vi "VMUI.vi"(10 "SubPanelRef":refnum<vi>, 11 "VariableManagerRef in":refnum<vi>) -> (3 "VariableManagerRef out":refnum<vi>)   [LabVIEW 2013]
doc: "The main user interface for VariableManager."
uses:
  VariableManager/VariableManager.lvclass
  VMUI.lvclass
  <vilib>/Utility/miscctls.llb/LVRowAndColumnUnsignedTypeDef.ctl
  SetListPrefs/SetListPrefs.lvclass/SetListPrefs.ctl
  <vilib>/Utility/miscctls.llb/LVRowAndColumnTypeDef.ctl
  Globals/PrefsGlobal.vi
  API/VariableManagerAPI.lvlib
  SetListPrefs/SetListPrefs.lvclass
panel:
  in  "VMUI":refnum<class "VMUI.lvclass">
  in  "Delete Variable":bool
  in  "Add Variable":bool
  in  "Edit Group":bool
  in  "Variable Group":u16(ring) items=["All"]
  in  "Detach":bool
  in  "Variables":string[][](table)
  in  "EvaluateSquenceValues":bool
  in  "Delete Sequence Index":bool
  in  "Add Sequence Index":bool
  in  "Sequence Indices":string[][](table)
  in  "Sequence Values":string[][](table) caption="Sequence Status"
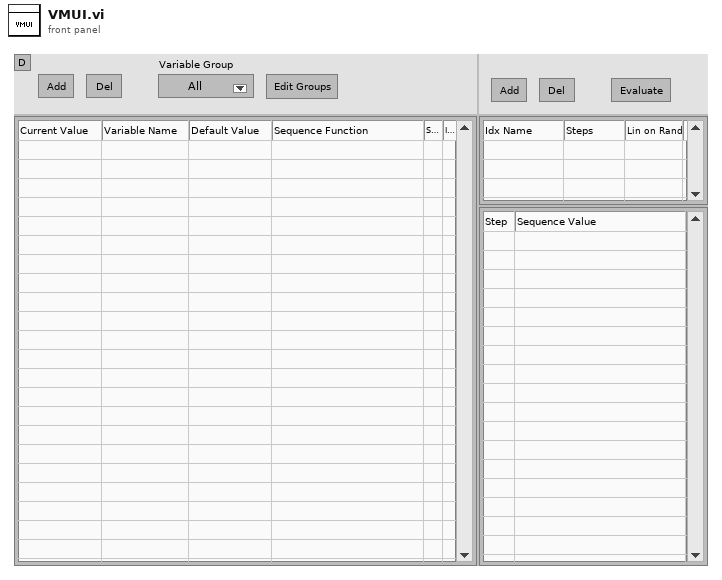
[diagram p1: front panel]
types:
  T1 = typedef "LVRowAndColumnUnsignedTypeDef.ctl" = cluster{"Row":u32, "Column":u32}
  T2 = typedef "LVRowAndColumnTypeDef.ctl" = cluster{"Row":i32, "Column":i32}
  T3 = cluster{"CtlRef":refnum<vi>, "OldVal":string[][], "NewVal":string[][]}
  T4 = typedef "LVPoint32TypeDef.ctl" = cluster{"Horizontal":i32, "Vertical":i32}
  T5 = cluster{"Shift":bool, "Ctrl":bool, "Alt":bool, "Cmd":bool, "Opt":bool}
  T6 = cluster{"CtlRef":refnum<vi>, "Coords":T4, "Button":u16, "Mods":cluster{"Double Click":bool, "Menu Key":bool}, "PlatMods":cluster{"Shift":bool, "Ctrl":bool, "Alt":bool, "Cmd":bool, "Opt":bool}}
  T7 = cluster{"Button":u16, "Mods":cluster{"Double Click":bool, "Menu Key":bool}, "PlatMods":cluster{"Shift":bool, "Ctrl":bool, "Alt":bool, "Cmd":bool, "Opt":bool}, "Discard?":bool}
  T8 = cluster{"CtlRef":refnum<vi>, "MenuRef":refnum<k9>, "Coords":T4, "SubObj":refnum<vi>}
  T9 = typedef "LVRectTypeDef.ctl" = cluster{"Left":i16, "Top":i16, "Right":i16, "Bottom":i16}
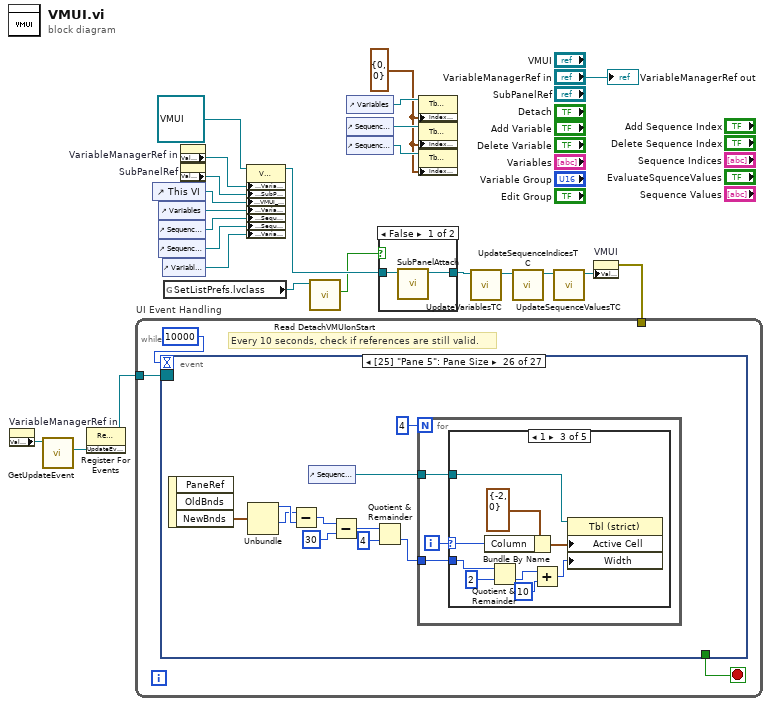
[diagram p0: block diagram]
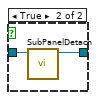
[diagram p2: hidden frame]
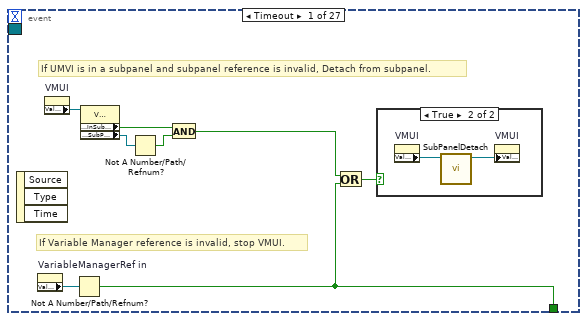
[diagram p3: hidden frame]
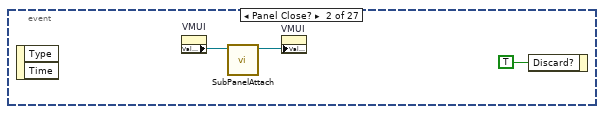
[diagram p5: hidden frame]
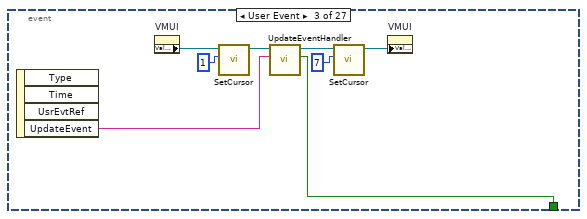
[diagram p6: hidden frame]
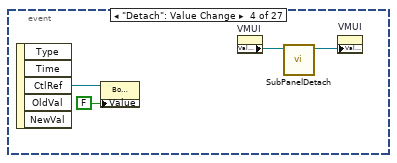
[diagram p7: hidden frame]
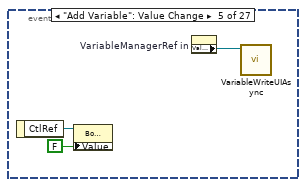
[diagram p8: hidden frame]
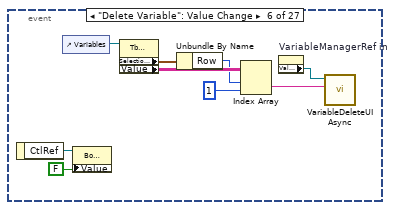
[diagram p9: hidden frame]
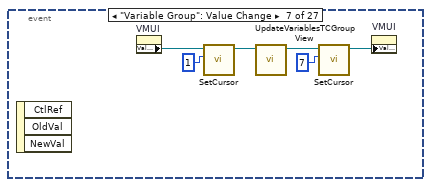
[diagram p10: hidden frame]
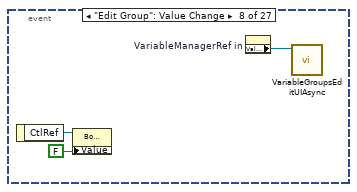
[diagram p11: hidden frame]
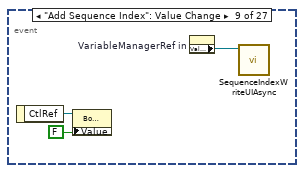
[diagram p12: hidden frame]
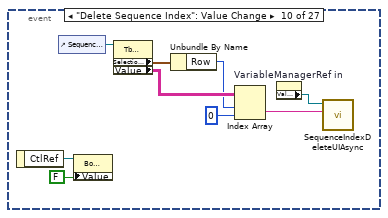
[diagram p13: hidden frame]
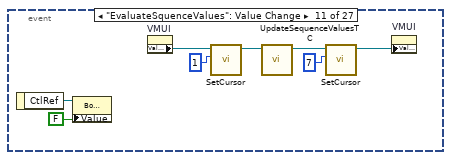
[diagram p14: hidden frame]
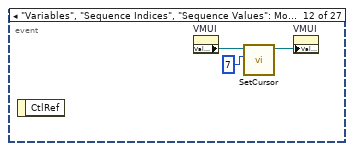
[diagram p15: hidden frame]
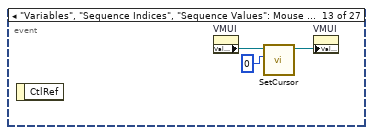
[diagram p16: hidden frame]
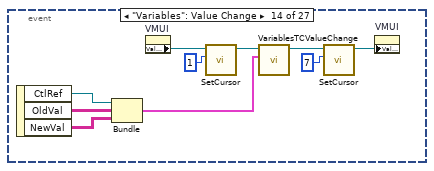
[diagram p17: hidden frame]
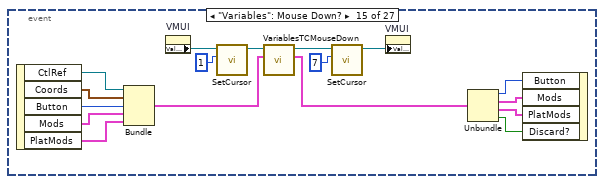
[diagram p18: hidden frame]
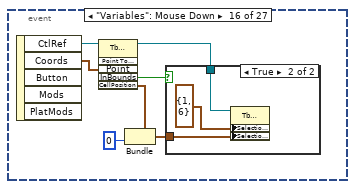
[diagram p19: hidden frame]
diagram:
  w4 = T1 {"Row"=0, "Column"=0} ("Index Values")
  n1 = property on="VariableManagerRef in" class="LVObjRef (strict)"() -> ("Value"=w15:refnum<vi>)  [unwired: 2 in, 2 out]
  n2 = call "GetUpdateEvent.vi"("VariableManagerRef in"=w15) -> ("UpdateEvent"=w14:refnum<user-event>)  [unwired: 8 in, 2 out]
  n3 = register-events(w14) -> (reference out=w13:refnum<event-registration>)  [unwired: 2 in, 1 out]
  n4 = control-ref of="This VI"() -> (w20:refnum<vi>)
  n5 = control-ref of="Variables"() -> (w19:refnum<vi>)
  n6 = control-ref of="Sequence Indices"() -> (w18:refnum<vi>)
  n7 = control-ref of="Sequence Values"() -> (w17:refnum<vi>)
  n8 = control-ref of="Variable Group"() -> (w16:refnum<vi>)
  n9 = global read "PrefsGlobal.vi" "SetListPrefs.lvclass"() -> (w2:refnum<class "SetListPrefs.lvclass">)
  n10 = property on="VariableManagerRef in" class="LVObjRef (strict)"() -> ("Value"=w22:refnum<vi>)  [unwired: 2 in, 2 out]
  n11 = property on="SubPanelRef" class="LVObjRef (strict)"() -> ("Value"=w21:refnum<vi>)  [unwired: 2 in, 2 out]
  n12 = property class="VMUI.lvclass"(reference=refnum<class "VMUI.lvclass"> refnum ("VMUI.lvclass"), "Accessors:VariableManagerRef"=w22, "Accessors:SubPanelRef"=w21, "Accessors:VMUI_VI_Ref"=w20, "Accessors:VariablesTCRef"=w19, "Accessors:SequenceIndicesTCRef"=w18, "Accessors:SequenceValuesTCRef"=w17, "Accessors:VariableGroupRingRef"=w16) -> (reference out=w12:refnum<class "VMUI.lvclass">)  [unwired: 1 in, 1 out]
  n13 = call "Read DetachVMUIonStart.vi"("SetListPrefs in"=w2) -> ("DetachVMUIonStart"=w1:bool)  [unwired: 8 in, 2 out]
  n14 = control-ref of="Variables"() -> (w7:refnum<vi>)
  n15 = control-ref of="Sequence Indices"() -> (w5:refnum<vi>)
  n16 = control-ref of="Sequence Values"() -> (w6:refnum<vi>)
  n17 = case shown="False" w1 {
    tunnel: w12 -> [w26 w27]
    tunnel: [w25 w28] -> w11
    frame False {
      n18 = call-dynamic "SubPanelAttach.vi"("VMUI in"=w26) -> ("VMUI out"=w25:refnum<class "VMUI.lvclass">)  [unwired: 9 in, 1 out]
    }
    frame True {
      n19 = call-dynamic "SubPanelDetach.vi"("VMUI in"=w27) -> ("VMUI out"=w28:refnum<class "VMUI.lvclass">)  [unwired: 9 in, 1 out]
    }
  }
  n20 = property class="Tbl (strict)"(reference=w7, "Index Values"=w4) -> ()  [unwired: 1 in, 2 out]
  n21 = property class="Tbl (strict)"(reference=w5, "Index Values"=w4) -> ()  [unwired: 1 in, 2 out]
  n22 = property class="Tbl (strict)"(reference=w6, "Index Values"=w4) -> ()  [unwired: 1 in, 2 out]
  n23 = call-dynamic "UpdateVariablesTC.vi"("VMUI in"=w11) -> ("VMUI out"=w10:refnum<class "VMUI.lvclass">)  [unwired: 9 in, 1 out]
  n24 = call-dynamic "UpdateSequenceIndicesTC.vi"("VMUI in"=w10) -> ("VMUI out"=w9:refnum<class "VMUI.lvclass">)  [unwired: 9 in, 1 out]
  n25 = call-dynamic "UpdateSequenceValuesTC.vi"("VMUI in"=w9) -> ("VMUI out"=w8:refnum<class "VMUI.lvclass">)  [unwired: 9 in, 1 out]
  n26 = property on="VMUI" class="LVClassControl (strict)"("Value"=w8) -> (error out=w3:errorcluster)  [unwired: 2 in, 1 out]
  n27 = while "UI Event Handling" {
    tunnel: w13 -> [w31]
    tunnel: w3 -> [_]
    stop <- w30 stop-if-true
    # "Every 10 seconds, check if references are still valid."
    n28 = event shown="[25] \"Pane 5\": Pane Size" {
      selector: w31 -> [_ _ _ _ _ _ _ _ _ _ _ _ _ _ _ _ _ _ _ _ _ _ _ _ _ _ _]
      dyn-events: _ -> [_ _ _ _ _ _ _ _ _ _ _ _ _ _ _ _ _ _ _ _ _ _ _ _ _ _ _]
      timeout: 10000 -> [_ _ _ _ _ _ _ _ _ _ _ _ _ _ _ _ _ _ _ _ _ _ _ _ _ _ _]
      tunnel: [w32 _ w51 _ _ _ _ _ _ _ _ _ _ _ _ _ _ _ _ _ _ _ _ _ _ _ _] -> w30
      event Timeout {
        # "If UMVI is in a subpanel and subpanel reference is invalid, Detach from subpanel."
        # "If Variable Manager reference is invalid, stop VMUI."
        n29 = event-data() -> ()  [unwired: 1 in, 3 out]
        n30 = property on="VariableManagerRef in" class="LVObjRef (strict)"() -> ("Value"=w39:refnum<vi>)  [unwired: 2 in, 2 out]
        n31 = property on="VMUI" class="LVClassControl (strict)"() -> ("Value"=w38:refnum<class "VMUI.lvclass">)  [unwired: 2 in, 2 out]
        n32 = Not A Number/Path/Refnum?(number/path/refnum=w39) -> (NaN/Path/Refnum?=w32:bool)
        n33 = property class="VMUI.lvclass"(reference=w38) -> ("Accessors:InSubPanel"=w36:bool, "Accessors:SubPanelRef"=w37:refnum<vi>)  [unwired: 1 in, 2 out]
        n34 = Not A Number/Path/Refnum?(number/path/refnum=w37) -> (NaN/Path/Refnum?=w35:bool)
        n35 = And(x=w36, y=w35) -> (x .and. y?=w33:bool)
        n36 = Or(x=w33, y=w32) -> (x .or. y?=w34:bool)
        n37 = case shown="True" w34 {
          frame False {
          }
          frame True {
            n38 = property on="VMUI" class="LVClassControl (strict)"() -> ("Value"=w41:refnum<class "VMUI.lvclass">)  [unwired: 2 in, 2 out]
            n39 = call-dynamic "SubPanelDetach.vi"("VMUI in"=w41) -> ("VMUI out"=w40:refnum<class "VMUI.lvclass">)  [unwired: 9 in, 1 out]
            n40 = property on="VMUI" class="LVClassControl (strict)"("Value"=w40) -> ()  [unwired: 2 in, 2 out]
          }
        }
      }
      event Panel Close? {
        n41 = event-data() -> ()  [unwired: 1 in, 2 out]
        n42 = property on="VMUI" class="LVClassControl (strict)"() -> ("Value"=w43:refnum<class "VMUI.lvclass">)  [unwired: 2 in, 2 out]
        n43 = call-dynamic "SubPanelAttach.vi"("VMUI in"=w43) -> ("VMUI out"=w42:refnum<class "VMUI.lvclass">)  [unwired: 9 in, 1 out]
        n44 = property on="VMUI" class="LVClassControl (strict)"("Value"=w42) -> ()  [unwired: 2 in, 2 out]
        n45 = event-data("Discard?"=TRUE) -> ()  [unwired: 1 in, 1 out]
      }
      event User Event {
        n46 = event-data() -> ("UpdateEvent"=w52:string)  [unwired: 1 in, 3 out]
        n47 = property on="VMUI" class="LVClassControl (strict)"() -> ("Value"=w48:refnum<class "VMUI.lvclass">)  [unwired: 2 in, 2 out]
        n48 = call-dynamic "SetCursor.vi"("icon"=u16 1, "VMUI in"=w48) -> ("VMUI out"=w47:refnum<class "VMUI.lvclass">)  [unwired: 8 in, 1 out]
        n49 = call-dynamic "UpdateEventHandler.vi"("UpdateEvent"=w52, "VMUI in"=w47) -> ("Stop"=w51:bool, "VMUI out"=w46:refnum<class "VMUI.lvclass">)  [unwired: 7 in, 1 out]
        n50 = call-dynamic "SetCursor.vi"("icon"=u16 7, "VMUI in"=w46) -> ("VMUI out"=w45:refnum<class "VMUI.lvclass">)  [unwired: 8 in, 1 out]
        n51 = property on="VMUI" class="LVClassControl (strict)"("Value"=w45) -> ()  [unwired: 2 in, 2 out]
      }
      event "Detach": Value Change {
        n52 = event-data() -> ("CtlRef"=w55:refnum<vi>)  [unwired: 1 in, 4 out]
        n53 = property class="Bool (strict)"(reference=w55, "Value"=FALSE) -> ()  [unwired: 1 in, 2 out]
        n54 = property on="VMUI" class="LVClassControl (strict)"() -> ("Value"=w54:refnum<class "VMUI.lvclass">)  [unwired: 2 in, 2 out]
        n55 = call-dynamic "SubPanelDetach.vi"("VMUI in"=w54) -> ("VMUI out"=w53:refnum<class "VMUI.lvclass">)  [unwired: 9 in, 1 out]
        n56 = property on="VMUI" class="LVClassControl (strict)"("Value"=w53) -> ()  [unwired: 2 in, 2 out]
      }
      event "Add Variable": Value Change {
        n57 = event-data() -> ("CtlRef"=w59:refnum<vi>)  [unwired: 1 in]
        n58 = property class="Bool (strict)"(reference=w59, "Value"=FALSE) -> ()  [unwired: 1 in, 2 out]
        n59 = property on="VariableManagerRef in" class="LVObjRef (strict)"() -> ("Value"=w57:refnum<vi>)  [unwired: 2 in, 2 out]
        n60 = call "VariableWriteUIAsync.vi"("VariableManagerRef in"=w57) -> ()  [unwired: 11 in]
      }
      event "Delete Variable": Value Change {
        n61 = event-data() -> ("CtlRef"=w68:refnum<vi>)  [unwired: 1 in]
        n62 = control-ref of="Variables"() -> (w62:refnum<vi>)
        n63 = property class="Bool (strict)"(reference=w68, "Value"=FALSE) -> ()  [unwired: 1 in, 2 out]
        n64 = property class="Tbl (strict)"(reference=w62) -> ("Selection Start"=w66:T2, "Value"=w65:string[][])  [unwired: 1 in, 2 out]
        n65 = Unbundle By Name(w66) -> ("Row"=w64:i32)
        n66 = Index Array(array=w65, index (row)=w64, index (col)=1 ("disabled index (col)")) -> (element=w60:string)
        n67 = property on="VariableManagerRef in" class="LVObjRef (strict)"() -> ("Value"=w61:refnum<vi>)  [unwired: 2 in, 2 out]
        n68 = call "VariableDeleteUIAsync.vi"("VariableName"=w60, "VariableManagerRef in"=w61) -> ()  [unwired: 10 in]
      }
      event "Variable Group": Value Change {
        n69 = event-data() -> ()  [unwired: 1 in, 3 out]
        n70 = property on="VMUI" class="LVClassControl (strict)"() -> ("Value"=w72:refnum<class "VMUI.lvclass">)  [unwired: 2 in, 2 out]
        n71 = call-dynamic "SetCursor.vi"("icon"=u16 1, "VMUI in"=w72) -> ("VMUI out"=w71:refnum<class "VMUI.lvclass">)  [unwired: 8 in, 1 out]
        n72 = call-dynamic "UpdateVariablesTCGroupView.vi"("VMUI in"=w71) -> ("VMUI out"=w70:refnum<class "VMUI.lvclass">)  [unwired: 9 in, 1 out]
        n73 = call-dynamic "SetCursor.vi"("icon"=u16 7, "VMUI in"=w70) -> ("VMUI out"=w69:refnum<class "VMUI.lvclass">)  [unwired: 8 in, 1 out]
        n74 = property on="VMUI" class="LVClassControl (strict)"("Value"=w69) -> ()  [unwired: 2 in, 2 out]
      }
      event "Edit Group": Value Change {
        n75 = event-data() -> ("CtlRef"=w77:refnum<vi>)  [unwired: 1 in]
        n76 = property class="Bool (strict)"(reference=w77, "Value"=FALSE) -> ()  [unwired: 1 in, 2 out]
        n77 = property on="VariableManagerRef in" class="LVObjRef (strict)"() -> ("Value"=w75:refnum<vi>)  [unwired: 2 in, 2 out]
        n78 = call "VariableGroupsEditUIAsync.vi"("VariableManagerRef in"=w75) -> ()  [unwired: 11 in]
      }
      event "Add Sequence Index": Value Change {
        n79 = event-data() -> ("CtlRef"=w80:refnum<vi>)  [unwired: 1 in]
        n80 = property class="Bool (strict)"(reference=w80, "Value"=FALSE) -> ()  [unwired: 1 in, 2 out]
        n81 = property on="VariableManagerRef in" class="LVObjRef (strict)"() -> ("Value"=w78:refnum<vi>)  [unwired: 2 in, 2 out]
        n82 = call "SequenceIndexWriteUIAsync.vi"("VariableManagerRef in"=w78) -> ()  [unwired: 11 in]
      }
      event "Delete Sequence Index": Value Change {
        n83 = event-data() -> ("CtlRef"=w89:refnum<vi>)  [unwired: 1 in]
        n84 = control-ref of="Sequence Indices"() -> (w83:refnum<vi>)
        n85 = property class="Bool (strict)"(reference=w89, "Value"=FALSE) -> ()  [unwired: 1 in, 2 out]
        n86 = property class="Tbl (strict)"(reference=w83) -> ("Selection Start"=w87:T2, "Value"=w86:string[][])  [unwired: 1 in, 2 out]
        n87 = Unbundle By Name(w87) -> ("Row"=w85:i32)
        n88 = Index Array(array=w86, index (row)=w85, index (col)=0 ("disabled index (col)")) -> (element=w81:string)
        n89 = property on="VariableManagerRef in" class="LVObjRef (strict)"() -> ("Value"=w82:refnum<vi>)  [unwired: 2 in, 2 out]
        n90 = call "SequenceIndexDeleteUIAsync.vi"("SequenceIndexName"=w81, "VariableManagerRef in"=w82) -> ()  [unwired: 10 in]
      }
      event "EvaluateSquenceValues": Value Change {
        n91 = event-data() -> ("CtlRef"=w97:refnum<vi>)  [unwired: 1 in]
        n92 = property class="Bool (strict)"(reference=w97, "Value"=FALSE) -> ()  [unwired: 1 in, 2 out]
        n93 = property on="VMUI" class="LVClassControl (strict)"() -> ("Value"=w93:refnum<class "VMUI.lvclass">)  [unwired: 2 in, 2 out]
        n94 = call-dynamic "SetCursor.vi"("icon"=u16 1, "VMUI in"=w93) -> ("VMUI out"=w92:refnum<class "VMUI.lvclass">)  [unwired: 8 in, 1 out]
        n95 = call-dynamic "UpdateSequenceValuesTC.vi"("VMUI in"=w92) -> ("VMUI out"=w91:refnum<class "VMUI.lvclass">)  [unwired: 9 in, 1 out]
        n96 = call-dynamic "SetCursor.vi"("icon"=u16 7, "VMUI in"=w91) -> ("VMUI out"=w90:refnum<class "VMUI.lvclass">)  [unwired: 8 in, 1 out]
        n97 = property on="VMUI" class="LVClassControl (strict)"("Value"=w90) -> ()  [unwired: 2 in, 2 out]
      }
      event "Variables", "Sequence Indices", "Sequence Values": Mouse Enter {
        n98 = event-data() -> ()  [unwired: 1 in, 1 out]
        n99 = property on="VMUI" class="LVClassControl (strict)"() -> ("Value"=w100:refnum<class "VMUI.lvclass">)  [unwired: 2 in, 2 out]
        n100 = call-dynamic "SetCursor.vi"("icon"=u16 7, "VMUI in"=w100) -> ("VMUI out"=w99:refnum<class "VMUI.lvclass">)  [unwired: 8 in, 1 out]
        n101 = property on="VMUI" class="LVClassControl (strict)"("Value"=w99) -> ()  [unwired: 2 in, 2 out]
      }
      event "Variables", "Sequence Indices", "Sequence Values": Mouse Leave {
        n102 = event-data() -> ()  [unwired: 1 in, 1 out]
        n103 = property on="VMUI" class="LVClassControl (strict)"() -> ("Value"=w103:refnum<class "VMUI.lvclass">)  [unwired: 2 in, 2 out]
        n104 = call-dynamic "SetCursor.vi"("icon"=u16 0, "VMUI in"=w103) -> ("VMUI out"=w102:refnum<class "VMUI.lvclass">)  [unwired: 8 in, 1 out]
        n105 = property on="VMUI" class="LVClassControl (strict)"("Value"=w102) -> ()  [unwired: 2 in, 2 out]
      }
      event "Variables": Value Change {
        n106 = event-data() -> ("CtlRef"=w113:refnum<vi>, "OldVal"=w112:string[][], "NewVal"=w111:string[][])  [unwired: 1 in]
        n107 = Bundle("CtlRef"=w113, "OldVal"=w112, "NewVal"=w111) -> (w110:T3)  [unwired: 1 in]
        n108 = property on="VMUI" class="LVClassControl (strict)"() -> ("Value"=w109:refnum<class "VMUI.lvclass">)  [unwired: 2 in, 2 out]
        n109 = call-dynamic "SetCursor.vi"("icon"=u16 1, "VMUI in"=w109) -> ("VMUI out"=w108:refnum<class "VMUI.lvclass">)  [unwired: 8 in, 1 out]
        n110 = call-dynamic "VariablesTCValueChange.vi"("ValueChangeIn"=w110, "VMUI in"=w108) -> ("VMUI out"=w107:refnum<class "VMUI.lvclass">)  [unwired: 8 in, 1 out]
        n111 = call-dynamic "SetCursor.vi"("icon"=u16 7, "VMUI in"=w107) -> ("VMUI out"=w106:refnum<class "VMUI.lvclass">)  [unwired: 8 in, 1 out]
        n112 = property on="VMUI" class="LVClassControl (strict)"("Value"=w106) -> ()  [unwired: 2 in, 2 out]
      }
      event "Variables": Mouse Down? {
        n113 = event-data() -> ("CtlRef"=w130:refnum<vi>, "Coords"=w129:T4, "Button"=w128:u16, "Mods"=w127:cluster{"Double Click":bool, "Menu Key":bool}, "PlatMods"=w126:T5)  [unwired: 1 in]
        n114 = Bundle("CtlRef"=w130, "Coords"=w129, "Button"=w128, "Mods"=w127, "PlatMods"=w126) -> (w114:T6)  [unwired: 1 in]
        n115 = property on="VMUI" class="LVClassControl (strict)"() -> ("Value"=w120:refnum<class "VMUI.lvclass">)  [unwired: 2 in, 2 out]
        n116 = call-dynamic "SetCursor.vi"("icon"=u16 1, "VMUI in"=w120) -> ("VMUI out"=w123:refnum<class "VMUI.lvclass">)  [unwired: 8 in, 1 out]
        n117 = call-dynamic "VariablesTCMouseDown.vi"("MouseDownIn"=w114, "VMUI in"=w123) -> ("MouseDownOut"=w119:T7, "VMUI out"=w122:refnum<class "VMUI.lvclass">)  [unwired: 7 in, 1 out]
        n118 = call-dynamic "SetCursor.vi"("icon"=u16 7, "VMUI in"=w122) -> ("VMUI out"=w121:refnum<class "VMUI.lvclass">)  [unwired: 8 in, 1 out]
        n119 = property on="VMUI" class="LVClassControl (strict)"("Value"=w121) -> ()  [unwired: 2 in, 2 out]
        n120 = Unbundle(w119) -> ("Button"=w118:u16, "Mods"=w117:cluster{"Double Click":bool, "Menu Key":bool}, "PlatMods"=w116:T5, "Discard?"=w115:bool)
        n121 = event-data("Button"=w118, "Mods"=w117, "PlatMods"=w116, "Discard?"=w115) -> ()  [unwired: 1 in, 1 out]
      }
      event "Variables": Mouse Down {
        n122 = event-data() -> ("CtlRef"=w137:refnum<vi>, "Coords"=w136:T4)  [unwired: 1 in, 3 out]
        n123 = invoke class="Tbl (strict)" method="Point To Row Column"(reference=w137, "Point"=w136) -> (reference out=w134:refnum<vi>, "InBounds"=w135:bool, "CellPosition"=w132:T2)  [unwired: 4 in, 3 out]
        n124 = Bundle(cluster=w132, "Column"=0) -> (w131:T2)  [unwired: 1 in]
        n125 = case shown="True" w135 {
          tunnel: w131 -> [_ w139]
          tunnel: w134 -> [_ w138]
          frame False {
          }
          frame True {
            n126 = property class="Tbl (strict)"(reference=w138, "Selection Size"=T2 {"Row"=1, "Column"=6}, "Selection Start"=w139) -> ()  [unwired: 1 in, 2 out]
          }
        }
      }
      event "Variables": Shortcut Menu Activation? {
        n127 = event-data() -> ("CtlRef"=w152:refnum<vi>, "MenuRef"=w151:refnum<k9>, "Coords"=w150:T4, "SubObj"=w149:refnum<vi>)  [unwired: 1 in]
        n128 = Bundle("CtlRef"=w152, "MenuRef"=w151, "Coords"=w150, "SubObj"=w149) -> (w144:T8)  [unwired: 1 in]
        n129 = property on="VMUI" class="LVClassControl (strict)"() -> ("Value"=w142:refnum<class "VMUI.lvclass">)  [unwired: 2 in, 2 out]
        n130 = call-dynamic "SetCursor.vi"("icon"=u16 1, "VMUI in"=w142) -> ("VMUI out"=w146:refnum<class "VMUI.lvclass">)  [unwired: 8 in, 1 out]
        n131 = call-dynamic "VariablesTCShortcutMenuCreate.vi"("ShortcutMenuIn"=w144, "VMUI in"=w146) -> ("Discard?"=w143:bool, "VMUI out"=w145:refnum<class "VMUI.lvclass">)  [unwired: 7 in, 1 out]
        n132 = call-dynamic "SetCursor.vi"("icon"=u16 7, "VMUI in"=w145) -> ("VMUI out"=w141:refnum<class "VMUI.lvclass">)  [unwired: 8 in, 1 out]
        n133 = property on="VMUI" class="LVClassControl (strict)"("Value"=w141) -> ()  [unwired: 2 in, 2 out]
        n134 = event-data("Discard?"=w143) -> ()  [unwired: 1 in, 1 out]
      }
      event "Variables": Shortcut Menu Selection (User) {
        n135 = event-data() -> ("CtlRef"=w156:refnum<vi>, "ItemTag"=w153:string, "ItemPath"=w154:string)  [unwired: 1 in, 2 out]
        n136 = property on="VariableManagerRef in" class="LVObjRef (strict)"() -> ("Value"=w155:refnum<vi>)  [unwired: 2 in, 2 out]
        n137 = case shown="Default" w154 {
          tunnel: w156 -> [_ w164 w173]
          tunnel: w155 -> [w157 w159 _]
          tunnel: w153 -> [_ _ w165]
          frame "Add" {
            n138 = call "VariableWriteUIAsync.vi"("VariableManagerRef in"=w157) -> ()  [unwired: 11 in]
          }
          frame "Delete" {
            n139 = property class="Tbl (strict)"(reference=w164) -> ("Value"=w163:string[][], "Selection Start"=w162:T2)  [unwired: 1 in, 2 out]
            n140 = Unbundle(w162) -> ("Row"=w161:i32)  [unwired: 1 out]
            n141 = Index Array(array=w163, index (row)=w161, index (col)=1 ("disabled index (col)")) -> (element=w158:string)
            n142 = call "VariableDeleteUIAsync.vi"("VariableName"=w158, "VariableManagerRef in"=w159) -> ()  [unwired: 10 in]
          }
          frame Default {
            # "Toggle variable's group"
            n143 = property class="Tbl (strict)"(reference=w173) -> ("Value"=w177:string[][], "Selection Start"=w176:T2)  [unwired: 1 in, 2 out]
            n144 = Unbundle(w176) -> ("Row"=w175:i32)  [unwired: 1 out]
            n145 = property on="VMUI" class="LVClassControl (strict)"() -> ("Value"=w170:refnum<class "VMUI.lvclass">)  [unwired: 2 in, 2 out]
            n146 = Index Array(array=w177, index (row)=w175, index (col)=1 ("disabled index (col)")) -> (element=w166:string)
            n147 = call-dynamic "SetCursor.vi"("icon"=u16 1, "VMUI in"=w170) -> ("VMUI out"=w168:refnum<class "VMUI.lvclass">)  [unwired: 8 in, 1 out]
            n148 = call-dynamic "VariableGroupToggle.vi"("GroupName"=w165, "VariableName"=w166, "VMUI in"=w168) -> ("VMUI out"=w167:refnum<class "VMUI.lvclass">)  [unwired: 7 in, 1 out]
            n149 = call-dynamic "SetCursor.vi"("icon"=u16 7, "VMUI in"=w167) -> ("VMUI out"=w169:refnum<class "VMUI.lvclass">)  [unwired: 8 in, 1 out]
            n150 = property on="VMUI" class="LVClassControl (strict)"("Value"=w169) -> ()  [unwired: 2 in, 2 out]
          }
        }
      }
      event "Sequence Indices": Value Change {
        n151 = event-data() -> ("CtlRef"=w187:refnum<vi>, "OldVal"=w186:string[][], "NewVal"=w185:string[][])  [unwired: 1 in]
        n152 = Bundle("CtlRef"=w187, "OldVal"=w186, "NewVal"=w185) -> (w178:T3)  [unwired: 1 in]
        n153 = property on="VMUI" class="LVClassControl (strict)"() -> ("Value"=w182:refnum<class "VMUI.lvclass">)  [unwired: 2 in, 2 out]
        n154 = call-dynamic "SetCursor.vi"("icon"=u16 1, "VMUI in"=w182) -> ("VMUI out"=w180:refnum<class "VMUI.lvclass">)  [unwired: 8 in, 1 out]
        n155 = call-dynamic "SequenceIndicesTCValueChange.vi"("ValueChangeIn"=w178, "VMUI in"=w180) -> ("VMUI out"=w179:refnum<class "VMUI.lvclass">)  [unwired: 8 in, 1 out]
        n156 = call-dynamic "SetCursor.vi"("icon"=u16 7, "VMUI in"=w179) -> ("VMUI out"=w181:refnum<class "VMUI.lvclass">)  [unwired: 8 in, 1 out]
        n157 = property on="VMUI" class="LVClassControl (strict)"("Value"=w181) -> ()  [unwired: 2 in, 2 out]
      }
      event "Sequence Indices": Mouse Down? {
        n158 = event-data() -> ("CtlRef"=w204:refnum<vi>, "Coords"=w203:T4, "Button"=w202:u16, "Mods"=w201:cluster{"Double Click":bool, "Menu Key":bool}, "PlatMods"=w200:T5)  [unwired: 1 in]
        n159 = Bundle("CtlRef"=w204, "Coords"=w203, "Button"=w202, "Mods"=w201, "PlatMods"=w200) -> (w193:T6)  [unwired: 1 in]
        n160 = property on="VMUI" class="LVClassControl (strict)"() -> ("Value"=w197:refnum<class "VMUI.lvclass">)  [unwired: 2 in, 2 out]
        n161 = call-dynamic "SetCursor.vi"("icon"=u16 1, "VMUI in"=w197) -> ("VMUI out"=w195:refnum<class "VMUI.lvclass">)  [unwired: 8 in, 1 out]
        n162 = call-dynamic "SequenceIndicesTCMouseDown.vi"("MouseDownIn"=w193, "VMUI in"=w195) -> ("MouseDownOut"=w192:T7, "VMUI out"=w194:refnum<class "VMUI.lvclass">)  [unwired: 7 in, 1 out]
        n163 = call-dynamic "SetCursor.vi"("icon"=u16 7, "VMUI in"=w194) -> ("VMUI out"=w196:refnum<class "VMUI.lvclass">)  [unwired: 8 in, 1 out]
        n164 = property on="VMUI" class="LVClassControl (strict)"("Value"=w196) -> ()  [unwired: 2 in, 2 out]
        n165 = Unbundle(w192) -> ("Button"=w189:u16, "Mods"=w191:cluster{"Double Click":bool, "Menu Key":bool}, "PlatMods"=w190:T5, "Discard?"=w188:bool)
        n166 = event-data("Button"=w189, "Mods"=w191, "PlatMods"=w190, "Discard?"=w188) -> ()  [unwired: 1 in, 1 out]
      }
      event "Sequence Indices": Mouse Down {
        n167 = event-data() -> ("CtlRef"=w209:refnum<vi>, "Coords"=w208:T4)  [unwired: 1 in, 3 out]
        n168 = invoke class="Tbl (strict)" method="Point To Row Column"(reference=w209, "Point"=w208) -> (reference out=w210:refnum<vi>, "InBounds"=w211:bool, "CellPosition"=w207:T2)  [unwired: 4 in, 3 out]
        n169 = Bundle(cluster=w207, "Column"=0) -> (w205:T2)  [unwired: 1 in]
        n170 = case shown="True" w211 {
          tunnel: w205 -> [_ w213]
          tunnel: w210 -> [_ w212]
          frame False {
          }
          frame True {
            n171 = property class="Tbl (strict)"(reference=w212, "Selection Size"=T2 {"Row"=1, "Column"=2}, "Selection Start"=w213) -> ()  [unwired: 1 in, 2 out]
          }
        }
      }
      event "Sequence Indices": Shortcut Menu Activation? {
        n172 = event-data() -> ("CtlRef"=w226:refnum<vi>, "MenuRef"=w225:refnum<k9>, "Coords"=w224:T4, "SubObj"=w223:refnum<vi>)  [unwired: 1 in]
        n173 = Bundle("CtlRef"=w226, "MenuRef"=w225, "Coords"=w224, "SubObj"=w223) -> (w216:T8)  [unwired: 1 in]
        n174 = property on="VMUI" class="LVClassControl (strict)"() -> ("Value"=w220:refnum<class "VMUI.lvclass">)  [unwired: 2 in, 2 out]
        n175 = call-dynamic "SetCursor.vi"("icon"=u16 1, "VMUI in"=w220) -> ("VMUI out"=w218:refnum<class "VMUI.lvclass">)  [unwired: 8 in, 1 out]
        n176 = call-dynamic "SequenceIndicesTCShortcutMenuCreate.vi"("ShortcutMenuIn"=w216, "VMUI in"=w218) -> ("Discard?"=w215:bool, "VMUI out"=w217:refnum<class "VMUI.lvclass">)  [unwired: 7 in, 1 out]
        n177 = call-dynamic "SetCursor.vi"("icon"=u16 7, "VMUI in"=w217) -> ("VMUI out"=w219:refnum<class "VMUI.lvclass">)  [unwired: 8 in, 1 out]
        n178 = property on="VMUI" class="LVClassControl (strict)"("Value"=w219) -> ()  [unwired: 2 in, 2 out]
        n179 = event-data("Discard?"=w215) -> ()  [unwired: 1 in, 1 out]
      }
      event "Sequence Indices": Shortcut Menu Selection (User) {
        n180 = event-data() -> ("CtlRef"=w229:refnum<vi>, "ItemTag"=w228:string)  [unwired: 1 in, 3 out]
        n181 = property on="VariableManagerRef in" class="LVObjRef (strict)"() -> ("Value"=w227:refnum<vi>)  [unwired: 2 in, 2 out]
        n182 = case shown="\"Delete\"" w228 {
          tunnel: w229 -> [_ w237]
          tunnel: w227 -> [w230 w231]
          frame "Add", Default {
            n183 = call "SequenceIndexWriteUIAsync.vi"("VariableManagerRef in"=w230) -> ()  [unwired: 11 in]
          }
          frame "Delete" {
            n184 = property class="Tbl (strict)"(reference=w237) -> ("Value"=w236:string[][], "Selection Start"=w235:T2)  [unwired: 1 in, 2 out]
            n185 = Unbundle(w235) -> ("Row"=w234:i32)  [unwired: 1 out]
            n186 = Index Array(array=w236, index (row)=w234, index (col)=0 ("disabled index (col)")) -> (element=w232:string)
            n187 = call "SequenceIndexDeleteUIAsync.vi"("SequenceIndexName"=w232, "VariableManagerRef in"=w231) -> ()  [unwired: 10 in]
          }
        }
      }
      event "Sequence Values": Mouse Down? {
        w238 = T2 {"Row"=0, "Column"=0} ("Selection Start")
        n188 = event-data() -> ("CtlRef"=w246:refnum<vi>, "Coords"=w245:T4, "Button"=w242:u16)  [unwired: 1 in, 2 out]
        n189 = Not Equal?(x=w242, y=u16 1) -> (x != y?=w240:bool)
        n190 = invoke class="Tbl (strict)" method="Point To Row Column"(reference=w246, "Point"=w245) -> (reference out=w244:refnum<vi>, "InBounds"=w241:bool)  [unwired: 4 in, 4 out]
        n191 = Or(x=w241, y=w240) -> (x .or. y?=w239:bool)
        n192 = property class="Tbl (strict)"(reference=w244, "Selection Size"=w238, "Selection Start"=w238) -> ()  [unwired: 1 in, 2 out]
        n193 = event-data("Discard?"=w239) -> ()  [unwired: 4 in, 1 out]
      }
      event Pane Size {
        n194 = event-data() -> ("NewBnds"=w248:T9)  [unwired: 1 in, 2 out]
        n195 = Unbundle(w248) -> ("Left"=w250:i16, "Right"=w249:i16)  [unwired: 2 out]
        n196 = Subtract(x=w249, y=w250) -> (x-y=w252:i16)
        n197 = control-ref of="Variables"() -> (w247:refnum<vi>)
        n198 = Subtract(x=w252, y=i16 64) -> (x-y=w254:i16)
        n199 = Quotient & Remainder(x=w254, y=i16 5) -> (floor(x/y)=w256:i16)  [unwired: 1 out]
        n200 = for {
          N: 6 -> [_]
          tunnel: w256 -> [w258]
          tunnel: w247 -> [w257]
          i -> [w259]
          n201 = case shown="4, 5" w259 {
            selector: w259 -> [_ w263 w270 w275]
            tunnel: w258 -> [_ w261 w267 _]
            tunnel: w257 -> [_ w260 w268 w272]
            frame Default {
            }
            frame 0..2 {
              n202 = Bundle By Name(cluster=T2 {"Row"=-2, "Column"=0} ("Active Cell:Active Cell"), "Column"=w263) -> (w262:T2)
              n203 = property class="Tbl (strict)"(reference=w260, "Active Cell"=w262, "Width"=w261) -> ()  [unwired: 1 in, 2 out]
            }
            frame 3 {
              n204 = Bundle By Name(cluster=T2 {"Row"=-2, "Column"=0} ("Active Cell:Active Cell"), "Column"=w270) -> (w269:T2)
              n205 = Multiply(x=w267, y=i16 2) -> (x*y=w266:i16)
              n206 = property class="Tbl (strict)"(reference=w268, "Active Cell"=w269, "Width"=w266) -> ()  [unwired: 1 in, 2 out]
            }
            frame 4, 5 {
              n207 = Bundle By Name(cluster=T2 {"Row"=-2, "Column"=0} ("Active Cell:Active Cell"), "Column"=w275) -> (w274:T2)
              n208 = property class="Tbl (strict)"(reference=w272, "Active Cell"=w274, "Width"=u32 17 ("Active Cell:Cell Size:Width")) -> ()  [unwired: 1 in, 2 out]
            }
          }
        }
      }
      event Pane Size {
        n209 = event-data() -> ("NewBnds"=w278:T9)  [unwired: 1 in, 2 out]
        n210 = Unbundle(w278) -> ("Left"=w280:i16, "Right"=w279:i16)  [unwired: 2 out]
        n211 = Subtract(x=w279, y=w280) -> (x-y=w282:i16)
        n212 = control-ref of="Sequence Indices"() -> (w277:refnum<vi>)
        n213 = Subtract(x=w282, y=i16 30) -> (x-y=w284:i16)
        n214 = Quotient & Remainder(x=w284, y=i16 4) -> (floor(x/y)=w286:i16)  [unwired: 1 out]
        n215 = for {
          N: 4 -> [_]
          tunnel: w286 -> [w288]
          tunnel: w277 -> [w287]
          i -> [w289]
          n216 = case shown="1" w289 {
            selector: w289 -> [_ w295 w302 w309 w316]
            tunnel: w288 -> [_ w292 w301 w308 w315]
            tunnel: w287 -> [_ w293 w303 w310 w317]
            frame Default {
            }
            frame 0 {
              n217 = Bundle By Name(cluster=T2 {"Row"=-2, "Column"=0} ("Active Cell:Active Cell"), "Column"=w295) -> (w294:T2)
              n218 = Add(x=w292, y=i16 5) -> (x+y=w291:i16)
              n219 = property class="Tbl (strict)"(reference=w293, "Active Cell"=w294, "Width"=w291) -> ()  [unwired: 1 in, 2 out]
            }
            frame 1 {
              n220 = Bundle By Name(cluster=T2 {"Row"=-2, "Column"=0} ("Active Cell:Active Cell"), "Column"=w302) -> (w304:T2)
              n221 = Quotient & Remainder(x=w301, y=i16 2) -> (floor(x/y)=w299:i16)  [unwired: 1 out]
              n222 = Add(x=w299, y=i16 10) -> (x+y=w297:i16)
              n223 = property class="Tbl (strict)"(reference=w303, "Active Cell"=w304, "Width"=w297) -> ()  [unwired: 1 in, 2 out]
            }
            frame 2 {
              n224 = Bundle By Name(cluster=T2 {"Row"=-2, "Column"=0} ("Active Cell:Active Cell"), "Column"=w309) -> (w311:T2)
              n225 = Add(x=w308, y=i16 15) -> (x+y=w307:i16)
              n226 = property class="Tbl (strict)"(reference=w310, "Active Cell"=w311, "Width"=w307) -> ()  [unwired: 1 in, 2 out]
            }
            frame 3 {
              n227 = Bundle By Name(cluster=T2 {"Row"=-2, "Column"=0} ("Active Cell:Active Cell"), "Column"=w316) -> (w318:T2)
              n228 = Add(x=w315, y=i16 5) -> (x+y=w314:i16)
              n229 = property class="Tbl (strict)"(reference=w317, "Active Cell"=w318, "Width"=w314) -> ()  [unwired: 1 in, 2 out]
            }
          }
        }
      }
      event Pane Size {
        n230 = event-data() -> ("NewBnds"=w321:T9)  [unwired: 1 in, 2 out]
        n231 = Unbundle(w321) -> ("Left"=w323:i16, "Right"=w322:i16)  [unwired: 2 out]
        n232 = Subtract(x=w322, y=w323) -> (x-y=w325:i16)
        n233 = control-ref of="Sequence Values"() -> (w320:refnum<vi>)
        n234 = Subtract(x=w325, y=i16 60) -> (x-y=w327:i16)
        n235 = for {
          N: 2 -> [_]
          tunnel: w327 -> [w329]
          tunnel: w320 -> [w328]
          i -> [w330]
          n236 = case shown="Default" w330 {
            selector: w330 -> [_ w334 w339]
            tunnel: w329 -> [_ _ w336]
            tunnel: w328 -> [_ w332 w337]
            frame Default {
            }
            frame 0 {
              n237 = Bundle By Name(cluster=T2 {"Row"=-2, "Column"=0} ("Active Cell:Active Cell"), "Column"=w334) -> (w333:T2)
              n238 = property class="Tbl (strict)"(reference=w332, "Active Cell"=w333, "Width"=u32 30 ("Active Cell:Cell Size:Width")) -> ()  [unwired: 1 in, 2 out]
            }
            frame 1 {
              n239 = Bundle By Name(cluster=T2 {"Row"=-2, "Column"=0} ("Active Cell:Active Cell"), "Column"=w339) -> (w338:T2)
              n240 = property class="Tbl (strict)"(reference=w337, "Active Cell"=w338, "Width"=w336) -> ()  [unwired: 1 in, 2 out]
            }
          }
        }
      }
    }
  }
  "VariableManagerRef out" <- "VariableManagerRef in"
